vi "Simple Solenoid - SubVI.vi"() -> ()   [LabVIEW 2019]
uses:
  <vilib>/Rock Robotics/WPI/Solenoid/WPI_SolenoidValue.ctl
  <vilib>/Rock Robotics/WPI/Solenoid/WPI_SolenoidSetEnum.vi
  <vilib>/Rock Robotics/WPI/Solenoid/WPI_SolenoidOpenDouble.vi
  <vilib>/Rock Robotics/WPI/Solenoid/WPI_SolenoidChannel.ctl
panel:
  in  "stop":bool
  in  "Value to Write":bool
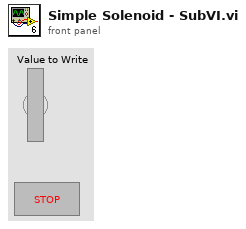
[diagram p1: front panel]
types:
  T1 = typedef "WPI_SolenoidChannel.ctl" = enum8{"Solenoid 0", "Solenoid 1", "Solenoid 2", "Solenoid 3", "Solenoid 4", "Solenoid 5", "Solenoid 6", "Solenoid 7", "Invalid"}
  T2 = typedef "WPI_SolenoidDevRef.ctl" = cluster{"DevStatus":errorcluster, "Pneumatics Control Module":u8, "Forward Solenoid Channel":T1, "Reverse Solenoid Channel":T1}
  T3 = typedef "WPI_SolenoidValue.ctl" = enum16{"Off", "On", "Forward", "Reverse"}
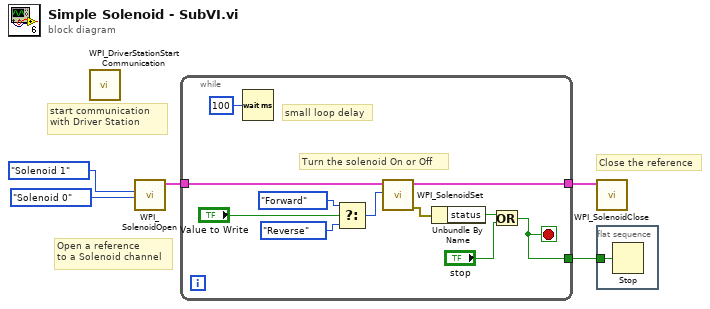
[diagram p0: block diagram]
diagram:
  # "start communication with Driver Station"
  # "Close the reference"
  # "Open a reference \nto a Solenoid channel"
  n1 = call <vilib>:"WPI_DriverStationStart Communication.vi"() -> ()  [unwired: 2 in, 10 out]
  n2 = call-poly <vilib>:"WPI_SolenoidOpen.vi"("Reverse Solenoid Channel"=WPI_SolenoidChannel."Solenoid 0", "Forward Solenoid Channel"=WPI_SolenoidChannel."Solenoid 1") -> ("SolenoidDevRef"=w5:T2)  [unwired: 2 in, 7 out]
  n3 = while {
    tunnel: w5 -> [w15]
    tunnel: [w14] -> w4
    tunnel: [w10] -> w3
    stop <- w10 stop-if-true
    # "small loop delay"
    # "Turn the solenoid On or Off"
    n4 = Wait (ms)(milliseconds to wait=u32 100) -> ()  [unwired: 1 out]
    n5 = Select(t=WPI_SolenoidValue."Forward" ("Value"), s="Value to Write", f=WPI_SolenoidValue."Reverse" ("Value")) -> (s? t:f=w6:T3)
    n6 = call-poly <vilib>:"WPI_SolenoidSet.vi"("Value"=w6, "SolenoidDevRef"=w15) -> ("error out"=w13:errorcluster, "SolenoidDevRef"=w14:T2)  [unwired: 1 in, 7 out]
    n7 = Unbundle By Name(w13) -> ("status"=w12:bool)
    n8 = Or(x=w12, y="stop") -> (x .or. y?=w10:bool)
  }
  n9 = call <vilib>:"WPI_SolenoidClose.vi"("SolenoidDevRef"=w4) -> ()  [unwired: 1 in, 10 out]
  n10 = flat-sequence {
    tunnel: w3 -> [w17]
    frame #0 {
      n11 = Stop(stop? (T)=w17) -> ()
    }
  }
